vi "CAL_PRESSURE_TRANSDUCER 2016.vi"(6 "Zero Pressure\n(F = leave as is)":bool=TRUE, 7 "Array in":refnum<k24>[](array[refnum]), 8 "error in (no error)":errorcluster, 9 "Descriptions":string[](array[string]), 10 "Sensor Cluster":T1, 11 "pressure_slope_IN":dbl=51.35 format="%.2f") -> (0 "error out":errorcluster, 2 "Sensor Cluster 2":T1, 3 "pressure_slope_OUT":dbl=51.35 format="%.2f", 5 "Array out":refnum<k24>[](array[refnum]))   [LabVIEW 2016]
uses:
  controls/MCC DAQ Readings.ctl
  C:/Cascade-lv16-64/builds/Waterloo Main Program/cascade/data/ULx_LV.dll
  builds/Waterloo Main Program/cascade/data/ULx_LV.dll
  Global_SIM_switch.vi
  Kpro Globals.vi
panel:
  out "Loop Counter":i32
  out "ok":bool
  out "zero":bool
  out "Pressure":dbl format="%.2f"
  in  "ok":bool
  in  "zero":bool
  # "PRESSURE TRANSDUCER CALIBRATION"
  # "(step 1)"
  # "Place graduated cylinder on floor.\nFill graduated cylinder to 750 mL water.\nSubmerge Kpro effluent and start flow.\nStop flow at 800 mL of water (1 foot).\nAllow pressure to equilibrate and press zero."
  # "(step 2)"
  # "Hold Kpro effluent facing up and 5' above the floor.\nTurn Kpro flow on briefly to fill the Kpro line.\nTurn Kpro flow off again.\nPress OK when pressure has equilibrated"
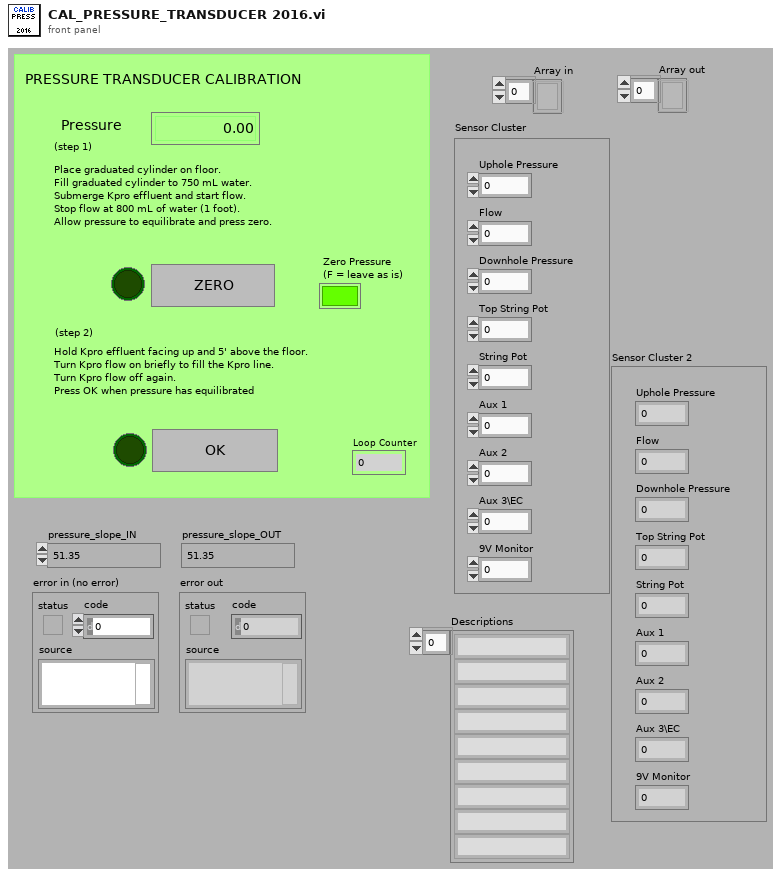
[diagram p1: front panel]
types:
  T1 = typedef "MCC DAQ Readings.ctl" = cluster{"Uphole Pressure":dbl, "Flow":dbl, "Downhole Pressure":dbl, "Top String Pot":dbl, "String Pot":dbl, "Aux 1":dbl, "Aux 2":dbl, "Aux 3\\EC":dbl, "9V Monitor":dbl}
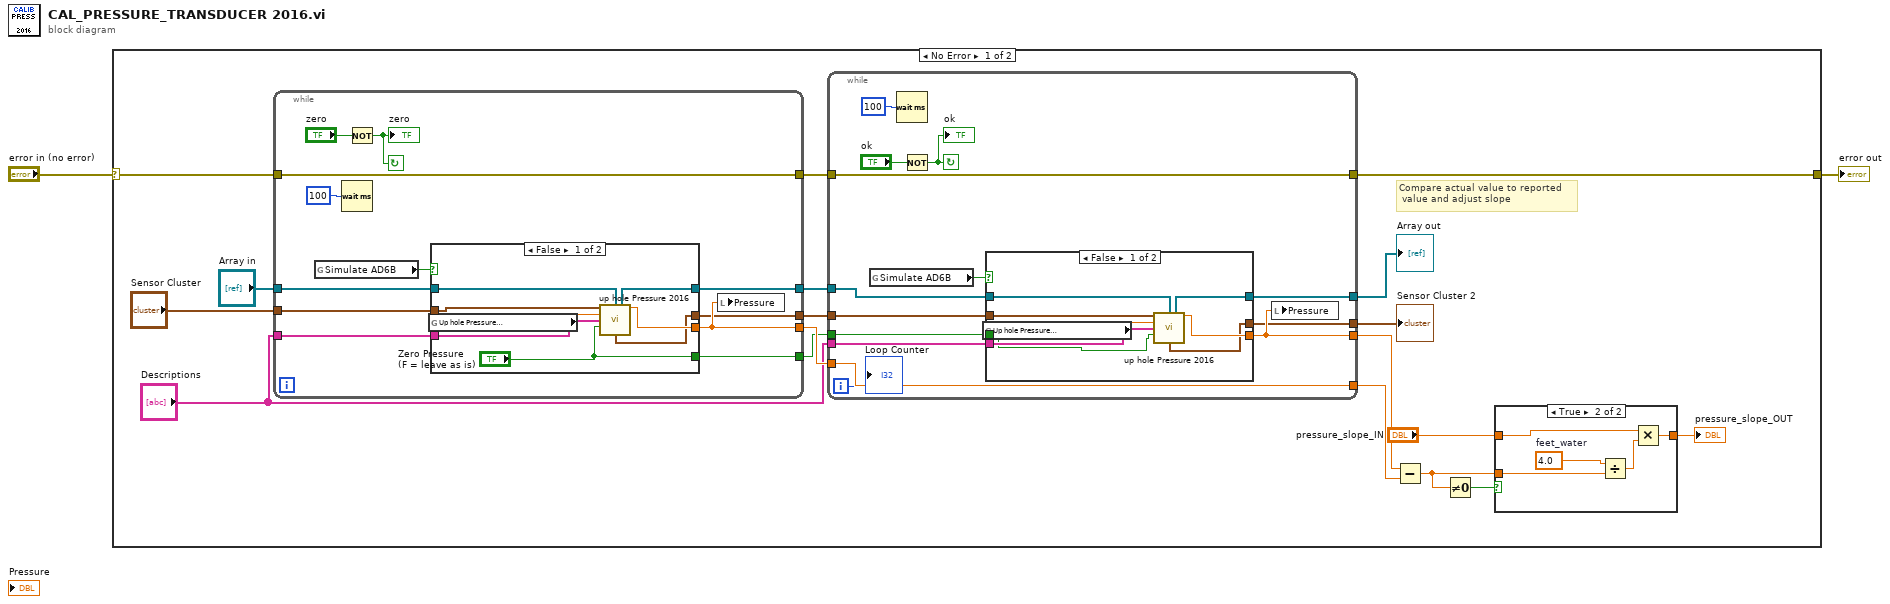
[diagram p0: block diagram]
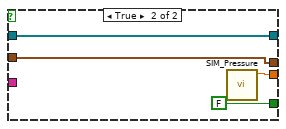
[diagram p3: hidden frame]
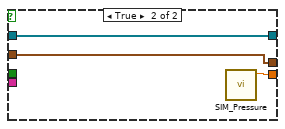
[diagram p4: hidden frame]
diagram:
  n1 = case shown="No Error" "error in (no error)" {
    selector: "error in (no error)" -> [w20 w76]
    tunnel: [w18 w76] -> w2
    frame No Error {
      # "Compare actual value to reported\n value and adjust slope"
      n2 = while {
        tunnel: [w35] -> w14
        tunnel: [w37] -> w19
        tunnel: w20 -> [w37]
        tunnel: "Sensor Cluster" -> [w32]
        tunnel: "Array in" -> [w31]
        tunnel: [w30] -> w12
        tunnel: "Descriptions" -> [w29]
        tunnel: [w28] -> w8
        tunnel: [w27] -> w3
        stop <- w33 continue-if-true
        n3 = global read "Global_SIM_switch.vi" "Simulate AD6B"() -> (w36:bool)
        n4 = Wait (ms)(milliseconds to wait=u32 100) -> ()  [unwired: 1 out]
        n5 = Not(x="zero") -> (.not. x?=w33:bool)
        "zero" <- w33
        n6 = case shown="False" w36 {
          tunnel: [w45 w50] -> w35
          tunnel: w32 -> [w46 w48]
          tunnel: w31 -> [w44 w49]
          tunnel: [w43 w49] -> w30
          tunnel: w29 -> [w42 _]
          tunnel: [w40 w48] -> w28
          tunnel: ["Zero Pressure\n(F = leave as is)" FALSE ("Zero Pressure\n(F = leave as is)")] -> w27
          frame False {
            n7 = global read "Kpro Globals.vi" "Up hole Pressure \nSlope"() -> (w41:dbl)
            n8 = call "up hole Pressure 2016.vi"("Sensor Cluster"=w46, "Array in"=w44, "Pressure \nSlope"=w41, "Descriptions"=w42, "Zero Pressure\n(F = leave as is)"="Zero Pressure\n(F = leave as is)") -> ("Array out"=w43:refnum<k24>[], "Uphole Pressure"=w45:dbl, "Sensor Cluster 2"=w40:T1)  [unwired: 7 in, 1 out]
          }
          frame True {
            n9 = call "SIM_Pressure.vi"() -> ("Pressure"=w50:dbl)  [unwired: 11 in]
          }
        }
        n10 = local write "Pressure"(w35) -> ()
      }
      n11 = while {
        tunnel: w14 -> [w62]
        tunnel: [w59] -> w15
        tunnel: [w62] -> w17
        tunnel: w19 -> [w63]
        tunnel: [w63] -> w18
        tunnel: w12 -> [w57]
        tunnel: [w56] -> w11
        tunnel: "Descriptions" -> [w55]
        tunnel: w8 -> [w54]
        tunnel: [w53] -> w7
        tunnel: w3 -> [w51]
        i -> [w52]
        stop <- w60 continue-if-true
        n12 = global read "Global_SIM_switch.vi" "Simulate AD6B"() -> (w58:bool)
        n13 = Wait (ms)(milliseconds to wait=u32 100) -> ()  [unwired: 1 out]
        n14 = Not(x="ok") -> (.not. x?=w60:bool)
        "ok" <- w60
        n15 = case shown="False" w58 {
          tunnel: [w71 w75] -> w59
          tunnel: w54 -> [w72 w73]
          tunnel: w57 -> [w70 w74]
          tunnel: [w69 w74] -> w56
          tunnel: w55 -> [w68 _]
          tunnel: [w66 w73] -> w53
          tunnel: w51 -> [w65 _]
          frame False {
            n16 = global read "Kpro Globals.vi" "Up hole Pressure \nSlope"() -> (w67:dbl)
            n17 = call "up hole Pressure 2016.vi"("Sensor Cluster"=w72, "Array in"=w70, "Pressure \nSlope"=w67, "Descriptions"=w68, "Zero Pressure\n(F = leave as is)"=w65) -> ("Array out"=w69:refnum<k24>[], "Uphole Pressure"=w71:dbl, "Sensor Cluster 2"=w66:T1)  [unwired: 7 in, 1 out]
          }
          frame True {
            n18 = call "SIM_Pressure.vi"() -> ("Pressure"=w75:dbl)  [unwired: 11 in]
          }
        }
        n19 = local write "Pressure"(w59) -> ()
        "Loop Counter" <- w52
      }
      "Array out" <- w11
      "Sensor Cluster 2" <- w7
      n20 = Subtract(x=w15, y=w17) -> (x-y=w6:dbl)
      n21 = Not Equal To 0?(x=w6) -> (x != 0?=w4:bool)
      n22 = case shown="True" w4 {
        tunnel: [w21 w25] -> w16
        tunnel: w6 -> [_ w23]
        tunnel: "pressure_slope_IN" -> [w21 w22]
        frame False {
        }
        frame True {
          w26 = 4.0  # feet_water
          n23 = Divide(x=w26, y=w23) -> (x/y=w24:dbl)
          n24 = Multiply(x=w22, y=w24) -> (x*y=w25:dbl)
        }
      }
      "pressure_slope_OUT" <- w16
    }
    frame Error {
    }
  }
  "error out" <- w2
